vi "Read Forward Drive State Ref.vi"(8 "error in (no error)":errorcluster, 11 "Logical Forward Drive in":refnum<class "Forward Drive.lvclass">) -> (0 "error out":errorcluster, 2 "Forward Drive State Ref":refnum<vi>, 3 "Logical Forward Drive out":refnum<class "Forward Drive.lvclass">)   [LabVIEW 2014, in "Forward Drive.lvlib" / "Forward Drive.lvclass"]
uses:
  Forward Drive.lvclass
  Virtual Robot/Virtual Forward Drive/Virtual Forward Drive Class/Forward Drive State.ctl
  Forward Drive.lvclass/Forward Drive.ctl
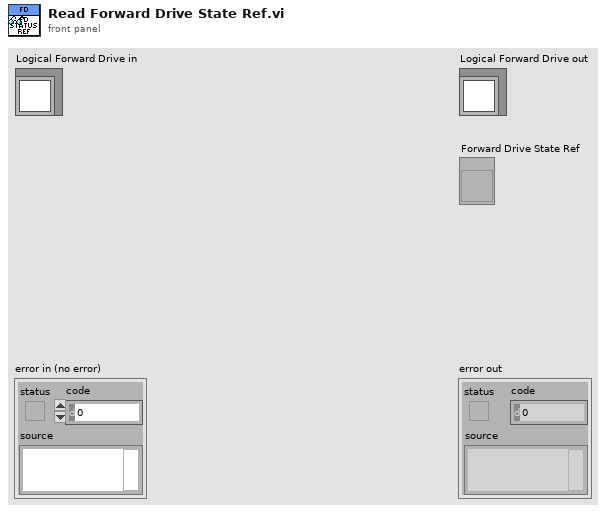
[diagram p1: front panel]
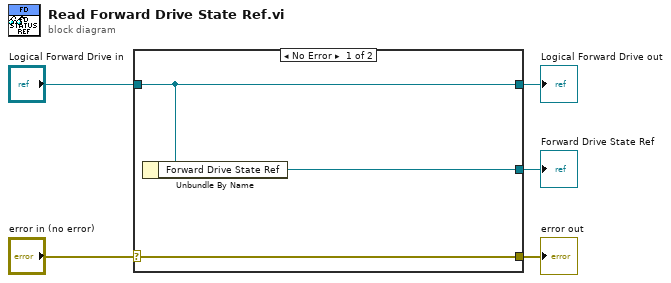
[diagram p0: block diagram]
diagram:
  n1 = case shown="No Error" "error in (no error)" {
    selector: "error in (no error)" -> [w8 w9]
    tunnel: [w8 w9] -> w4
    tunnel: [w7 w10] -> w2
    tunnel: "Logical Forward Drive in" -> [w7 w10]
    tunnel: [w6 _] -> w1
    frame No Error {
      n2 = Unbundle By Name(w7) -> ("Forward Drive State Ref"=w6:refnum<vi>)
    }
    frame Error {
    }
  }
  "error out" <- w4
  "Logical Forward Drive out" <- w2
  "Forward Drive State Ref" <- w1
